vi "Read ConfigInterface.vi"(11 "Proccess in":refnum<class "Proccess.lvclass">) -> (2 "ConfigInterface":refnum<class "ConfigInterface.lvclass">, 3 "Proccess out":refnum<class "Proccess.lvclass">)   [LabVIEW 2019, in "Proccess.lvclass"]
uses:
  Proccess.lvclass
  ConfigInterface_class/ConfigInterface.lvclass
  Proccess.lvclass/Proccess.ctl
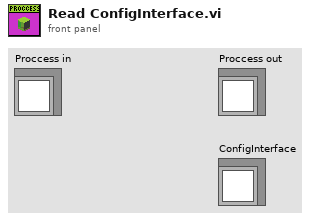
[diagram p1: front panel]
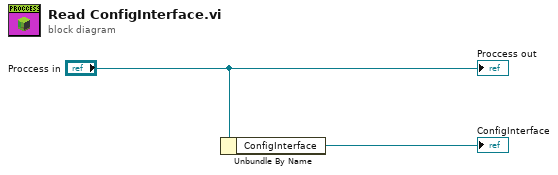
[diagram p0: block diagram]
diagram:
  n1 = Unbundle By Name("Proccess in") -> ("ConfigInterface"=→"ConfigInterface":refnum<class "ConfigInterface.lvclass">)
  "Proccess out" <- "Proccess in"
